vi "Seq Commands.vi"(11 "Loop Data in":T1) -> (3 "Loop Data":T1)   [LabVIEW 2020, in "VolatusDaq.lvlib" / "DaqControl.lvclass"]
uses:
  DaqControl.lvclass
  DaqControl.lvclass/DaqControl.ctl
  Value Update.ctl
  Sequence Action.ctl
  VolatusDaq.lvlib
  Loop Data.ctl
  Seq Cmd Type.ctl
  Seq Action Type.ctl
  Seq Cmd.ctl
  Signal Type.ctl
  Volatus/Event API/EventAPI.lvclass
  Volatus/DataHandlerAPI/DataHandlerAPI.lvclass
  Sequence.ctl
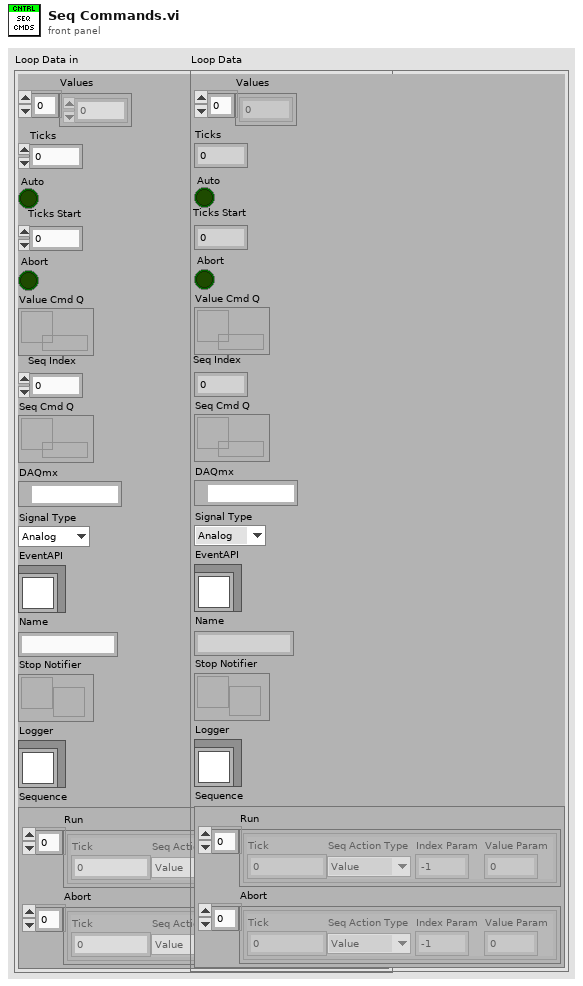
[diagram p1: front panel]
types:
  T1 = typedef "VolatusDaq.lvlib/DaqControl.lvclass/Loop Data.ctl" = cluster{"Values":dbl[], "Ticks":u32, "Auto":bool, "Ticks Start":u32, "Abort":bool, "Value Cmd Q":refnum<queue>, "Seq Index":i32, "Seq Cmd Q":refnum<queue>, "DAQmx":refnum<k21>, "Signal Type":T2, "EventAPI":refnum<class "EventAPI.lvclass">, "Name":string, "Stop Notifier":refnum<notifier>, "Logger":refnum<class "DataHandlerAPI.lvclass">, "Sequence":T3}
  T2 = typedef "VolatusDaq.lvlib/Signal Type.ctl" = enum16{"Analog", "Digital"}
  T3 = typedef "VolatusDaq.lvlib/Sequence.ctl" = cluster{"Run":T4[], "Abort":T4[]}
  T4 = typedef "VolatusDaq.lvlib/Sequence Action.ctl" = cluster{"Tick":u32, "Seq Action Type":T5, "Index Param":i32, "Value Param":dbl}
  T5 = typedef "VolatusDaq.lvlib/Seq Action Type.ctl" = enum16{"Value", "Stop"}
  T6 = typedef "VolatusDaq.lvlib/DaqControl.lvclass/Seq Cmd.ctl" = cluster{"Type":T7, "Seq Index":i32}
  T7 = typedef "VolatusDaq.lvlib/DaqControl.lvclass/Seq Cmd Type.ctl" = enum16{"Timeout", "Abort", "Reset Ticks", "Prepare", "Start"}
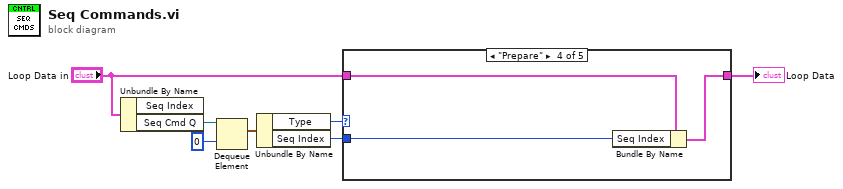
[diagram p0: block diagram]
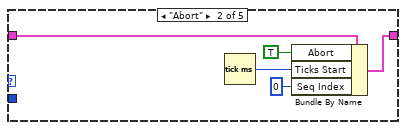
[diagram p3: hidden frame]
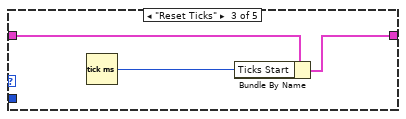
[diagram p4: hidden frame]
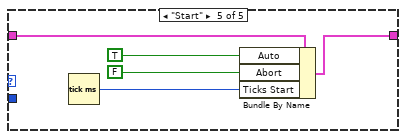
[diagram p5: hidden frame]
diagram:
  n1 = Unbundle By Name("Loop Data in") -> ("Seq Cmd Q"=w7:refnum<queue>)  [unwired: 1 out]
  n2 = Dequeue Element(queue=w7, timeout in ms (-1)=0) -> (element=w3:T6)  [unwired: 1 in, 3 out]
  n3 = Unbundle By Name(w3) -> ("Type"=w2:T7, "Seq Index"=w1:i32)
  n4 = case shown="\"Prepare\"" w2 {
    tunnel: "Loop Data in" -> [w8 w10 w16 w19 w24]
    tunnel: [w8 w11 w15 w18 w20] -> w4
    tunnel: w1 -> [_ _ _ w17 _]
    frame "Timeout" {
    }
    frame "Abort" {
      n5 = Tick Count (ms)() -> (millisecond timer value=w12:u32)
      n6 = Bundle By Name(cluster=w10, "Abort"=TRUE, "Ticks Start"=w12, "Seq Index"=0) -> (w11:T1)
    }
    frame "Reset Ticks" {
      n7 = Tick Count (ms)() -> (millisecond timer value=w14:u32)
      n8 = Bundle By Name(cluster=w16, "Ticks Start"=w14) -> (w15:T1)
    }
    frame "Prepare" {
      n9 = Bundle By Name(cluster=w19, "Seq Index"=w17) -> (w18:T1)
    }
    frame "Start" {
      n10 = Tick Count (ms)() -> (millisecond timer value=w21:u32)
      n11 = Bundle By Name(cluster=w24, "Auto"=TRUE, "Abort"=FALSE, "Ticks Start"=w21) -> (w20:T1)
    }
  }
  "Loop Data" <- w4
